vi "fraction to pulses.vi"(10 "fractions":dbl[](array[numeric])=[0.0001, 0.2, 0.49, 0.8, 0.9, 0.99, 0.999, 0.0, 0.0, 0.0, 0.0, 0.0, 0.2, 0.0, 0.0, 0.0]) -> (0 "error out":dbl[](array[numeric])=[0.0001, 0.2, 0.49, 0.8, 0.9, 0.99, 0.999], 1 "switch state":bool[](array[boolean]), 2 "pulses per cycle":u32[](array[numeric]), 3 "pulses on":u32[](array[numeric]), 4 "cycle length (s)":dbl[](array[numeric]), 5 "minimum pulse time (ms) 2":u32)   [LabVIEW 2012]
panel:
  out "Array":dbl[](array[numeric])
  in  "minimum pulse time (ms)":u32=50
  in  "minimum cycle time (ms)":u32=1000
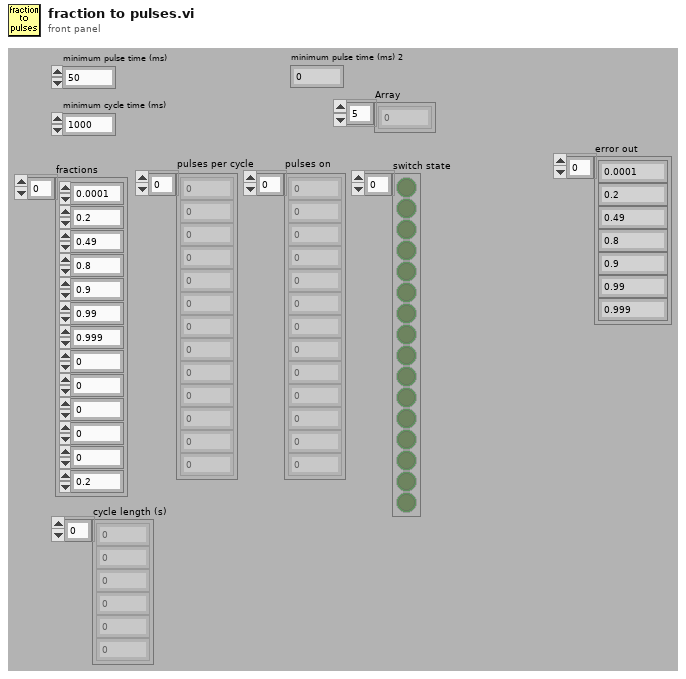
[diagram p1: front panel]
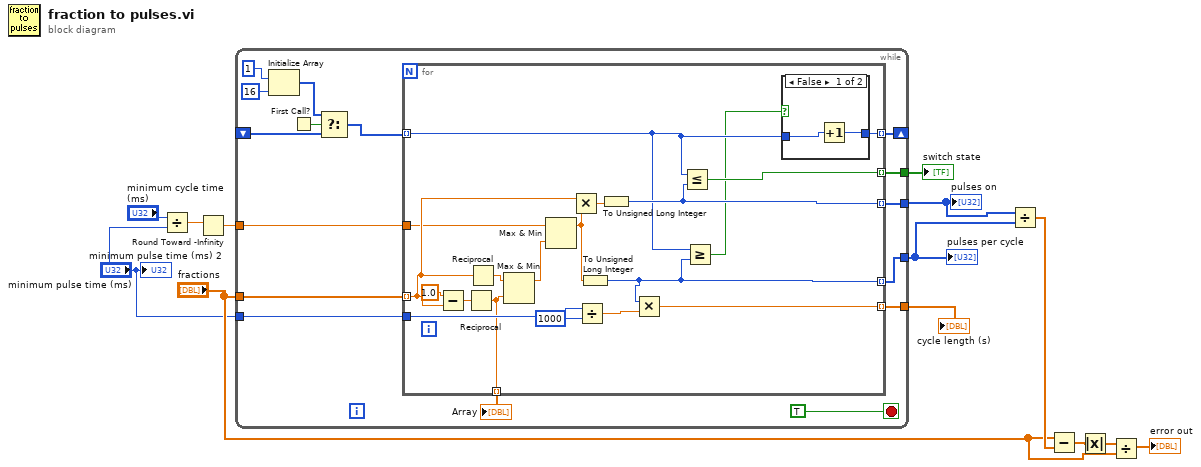
[diagram p0: block diagram]
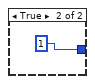
[diagram p2: hidden frame]
diagram:
  n1 = Divide(x="minimum cycle time (ms)", y="minimum pulse time (ms)") -> (x/y=w12:dbl)
  n2 = Round Toward -Infinity(1:w12) -> (0:w6:dbl)
  n3 = while {
    tunnel: "fractions" -> [w29]
    tunnel: w6 -> [w28]
    tunnel: [w27] -> w5
    tunnel: [w26] -> w4
    shift-right: [w24] -> _
    shift-left: _ -> [w22]
    tunnel: [w23] -> w3
    tunnel: "minimum pulse time (ms)" -> [w19]
    tunnel: [w18] -> w1
    stop <- TRUE stop-if-true
    n4 = Initialize Array(1, 16 ("dimension size")) -> (w15:i32[])
    n5 = First Call?() -> (First Call?: T/F=w20:bool)
    n6 = Select(t=w15, s=w20, f=w22) -> (s? t:f=w21:i32[])
    n7 = for {
      tunnel: w29 -> [w43] mode=indexing
      tunnel: [w35] -> w27 mode=indexing
      tunnel: [w40] -> w26 mode=indexing
      tunnel: w28 -> [w41]
      tunnel: [w39] -> w23 mode=indexing
      tunnel: [w38] -> w24 mode=indexing
      tunnel: w21 -> [w37] mode=indexing
      tunnel: w19 -> [w34]
      tunnel: [w33] -> w18 mode=indexing
      tunnel: [w30] -> w14 mode=indexing
      n8 = Subtract(x=1.0, y=w43) -> (x-y=w47:dbl)
      n9 = Reciprocal(x=w47) -> (1/x=w30:dbl)
      n10 = Reciprocal(x=w43) -> (1/x=w46:dbl)
      n11 = Max & Min(x=w46, y=w30) -> (max(x,y)=w45:dbl)  [unwired: 1 out]
      n12 = Max & Min(x=w41, y=w45) -> (max(x,y)=w44:dbl)  [unwired: 1 out]
      n13 = Multiply(x=w43, y=w44) -> (x*y=w42:dbl)
      n14 = Divide(x=w34, y=u32 1000) -> (x/y=w32:dbl)
      n15 = To Unsigned Long Integer(number=w44) -> (unsigned 32bit integer=w35:u32)
      n16 = To Unsigned Long Integer(number=w42) -> (unsigned 32bit integer=w40:u32)
      n17 = Multiply(x=w35, y=w32) -> (x*y=w33:dbl)
      n18 = Less Or Equal?(x=w37, y=w40) -> (x <= y?=w39:bool)
      n19 = Greater Or Equal?(x=w37, y=w35) -> (x >= y?=w36:bool)
      n20 = case shown="False" w36 {
        tunnel: [w50 1] -> w38
        tunnel: w37 -> [w49 _]
        frame False {
          n21 = Increment(x=w49) -> (x+1=w50:i32)
        }
        frame True {
        }
      }
    }
    "Array" <- w14
  }
  "pulses per cycle" <- w5
  "pulses on" <- w4
  "switch state" <- w3
  "cycle length (s)" <- w1
  n22 = Divide(x=w4, y=w5) -> (x/y=w11:dbl[])
  n23 = Subtract(x="fractions", y=w11) -> (x-y=w10:dbl[])
  n24 = Absolute Value(x=w10) -> (abs(x)=w7:dbl[])
  n25 = Divide(x=w7, y="fractions") -> (x/y=→"error out":dbl[])
  "minimum pulse time (ms) 2" <- "minimum pulse time (ms)"
